vi "MGI Validate Log Directory.vi"(10 "Log Directory (<Not a Path>: Use Default)":path, 11 "MGI Error Reporter In":refnum<class "MGI Error Reporter Base.lvclass">) -> (2 "Validated Path":path, 3 "MGI Error Reporter Out":refnum<class "MGI Error Reporter Base.lvclass">)   [LabVIEW 2020, in "MGI Error Reporter Base.lvclass"]
doc: "Validate the specified path, outputting a default path if the specified path is <Not a Path>.\n\nAuthored by Shawn Walpole\nsupport@mooregoodideas.com\nwww.mooregoodideas.com\n\nCopyright (c) 2013, Moore Good Ideas, Inc.\n\nAll rights reserved.\n\nRedistribution and use in source and binary forms, with or without modification, are permitted provided that the following conditions are met:\n\n * Redistributions of source code must retain the above copyright notice, this list of conditions and the following disclaimer.\n * Redistributions in binary form must reproduce the above copyright notice, this list of conditions and the following disclaimer in the documentation and/or other materials provided with the distribution.\n * Neither the name of Moore Good Ideas, Inc. nor the names of its contributors may be used to endorse or promote products derived from this software without specific prior written permission.\n\nTHIS SOFTWARE IS PROVIDED BY THE COPYRIGHT HOLDERS AND CONTRIBUTORS \"AS IS\" AND ANY EXPRESS OR IMPLIED WARRANTIES, INCLUDING, BUT NOT LIMITED TO, THE IMPLIED WARRANTIES OF MERCHANTABILITY AND FITNESS FOR A PARTICULAR PURPOSE ARE DISCLAIMED. IN NO EVENT SHALL THE COPYRIGHT OWNER OR CONTRIBUTORS BE LIABLE FOR ANY DIRECT, INDIRECT, INCIDENTAL, SPECIAL, EXEMPLARY, OR CONSEQUENTIAL DAMAGES (INCLUDING, BUT NOT LIMITED TO, PROCUREMENT OF SUBSTITUTE GOODS OR SERVICES; LOSS OF USE, DATA, OR PROFITS; OR BUSINESS INTERRUPTION) HOWEVER CAUSED AND ON ANY THEORY OF LIABILITY, WHETHER IN CONTRACT, STRICT LIABILITY, OR TORT (INCLUDING NEGLIGENCE OR OTHERWISE) ARISING IN ANY WAY OUT OF THE USE OF THIS SOFTWARE, EVEN IF ADVISED OF THE POSSIBILITY OF SUCH DAMAGE."
uses:
  <userlib>/_MGI/Error Reporter/MGI Error Reporter Base/MGI Error Reporter Base.lvclass
  <userlib>/_MGI/File/MGI Windows Folder Enum.ctl
  <userlib>/_MGI/Application Control/MGI VI Reference/MGI Top Level VI Reference.vi
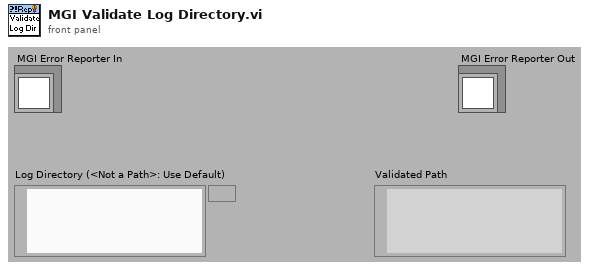
[diagram p1: front panel]
types:
  T1 = typedef "MGI Windows Folder Enum.ctl" = enum32{"Desktop", "Err<Internet>", "Programs", "Err<Controls>", "Err<Printers>", "Personal (MyDocuments)", "Favorites", "Startup", "Recent", "SendTo", "Err<RecycleBin>", "StartMenu", "Err<MyDocuments>", "MyMusic", "MyVideo", "Err<0x000F>", "DesktopDirectory", "Err<Drives>", "Err<Network>", "NetHood", "Fonts", "Templates", "CommonStartMenu", "CommonPrograms", "CommonStartup", "CommonDesktopDirectory", "AppData", "PrintHood", "LocalAppData", "Err<AltStartup>", "Err<CommonAltStartup>", "CommonFavorites", "InternetCache", "Cookies", "History", "CommonAppData", "Windows", "System", "ProgramFiles", "MyPictures", "Profile", "System32", "Err<0x002A>", "ProgramFilesCommon", "Err<0x002C>", "CommonTemplates", "CommonDocuments", "CommonAdminTools", "AdminTools"}
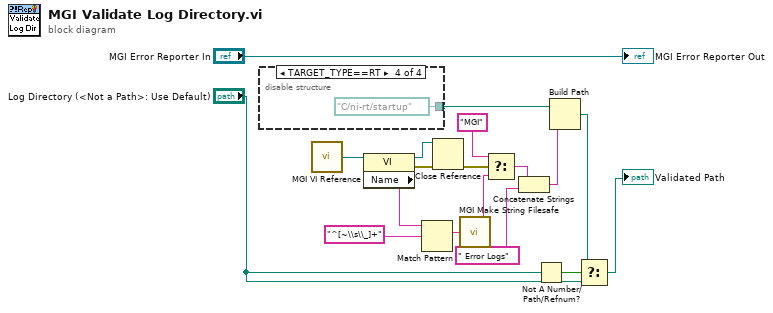
[diagram p0: block diagram]
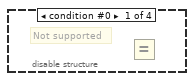
[diagram p2: hidden frame]
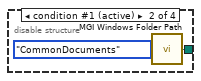
[diagram p3: hidden frame]
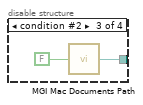
[diagram p4: hidden frame]
diagram:
  n1 = disable-structure shown="TARGET_TYPE==RT" {
    disable-tunnel: [_ w20 w22 path "C:/ni-rt/startup" ("Path")] -> w14
    frame condition #0 {
      # "Not supported"
      n2 = Equal?() -> ()  [unwired: 2 in, 1 out]
    }
    frame condition #1 (active) {
      n3 = call <userlib>:"MGI Windows Folder Path.vi"("Windows Folder"=MGI_Windows_Folder_Enum."CommonDocuments") -> ("Path"=w20:path)
    }
    frame condition #2 {
      n4 = call <userlib>:"MGI Mac Documents Path.vi"("User Documents? (F: Shared Documents)"=FALSE) -> ("Path"=w22:path)
    }
    frame condition #3 {
    }
  }
  n5 = call-poly <userlib>:"MGI VI Reference.vi"() -> ("Top Level VI Reference"=w13:refnum<vi>)  [unwired: 1 out]
  n6 = property class="VI"(reference=w13) -> (reference out=w11:refnum<vi>, error out=w12:errorcluster, "Name"=w7:string)  [unwired: 1 in]
  n7 = Match Pattern(string=w7, regular expression="^[~\\s\\_]+") -> (match substring=w5:string)  [unwired: 4 out]
  n8 = Close Reference(reference=w11, error in (no error)=w12) -> (error out=w10:errorcluster)
  n9 = call <userlib>:"MGI Make String Filesafe.vi"("String In"=w5) -> ("Filesafe String Out"=w4:string)
  n10 = Select(t="MGI", s=w10, f=w4) -> (s? t:f=w3:string)
  n11 = Concatenate Strings(w3, " Error Logs" ("string")) -> (w2:string)
  n12 = Not A Number/Path/Refnum?(number/path/refnum="Log Directory (<Not a Path>: Use Default)") -> (NaN/Path/Refnum?=w15:bool)
  n13 = Build Path(base path=w14, name or relative path=w2) -> (appended path=w9:path)
  n14 = Select(t=w9, s=w15, f="Log Directory (<Not a Path>: Use Default)") -> (s? t:f=→"Validated Path":path)
  "MGI Error Reporter Out" <- "MGI Error Reporter In"
